vi "OAT Easy Gabor Order Tracking.vi"   [LabVIEW 2017]
doc: "Extracts orders you designate from <B>scaled signal [EU]</B> and computes magnitudes and phase lags for the designated orders. You can use this polymorphic VI to perform order tracking for an analog tachometer signal or a digital tachometer signal. The data type you wire to the <B>analog tach signal</B> input determines the polymorphic instance to use."
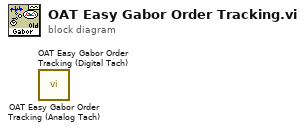
[diagram p0: block diagram]
diagram:
  n1 = call <vilib>:"OAT Easy Gabor Order Tracking (Analog Tach).vi"() -> ()  [unwired: 10 in, 6 out]
  n2 = call <vilib>:"OAT Easy Gabor Order Tracking (Digital Tach).vi"() -> ()  [unwired: 10 in, 6 out]
